vi "FaulhaberV3Communication.vi"(6 "Knoten":u8=1, 7 "Befehl":T1(ring)=enum."SDORead", 8 "error in (no error)":errorcluster, 9 "SendValue":u8[](array[numeric]) format="%02x", 10 "SendObject":u32=1614807040 format="%04x", 11 "VISA resource name":refnum<visa-resource-name>="COM10") -> (0 "error out":errorcluster={"status"=FALSE, "code"=1073676293, "source"="VISA Read in FaulhaberCommunication.vi->Faulhaber_Standalone.vi"}, 1 "Return Value":u8[](array[numeric]) format="%02x", 2 "RecieveObject":u32 format="%08x", 3 "VISA resource name out":refnum<visa-resource-name>="COM10")   [LabVIEW 2011]
panel:
  out "raw":cluster{"unsigned byte array":u8[]}[](array[cluster]) {"unsigned byte array" format="%02x"}
  out "ResponseNo":i32
  out "raw Response":u8[](array[numeric]) format="%02x"
  out "to send unsigned byte array":u8[](array[numeric])=[71, 65, 67, 13] format="%02x"
  out "Bytes send":u32=4
  # "2025 new binary interface"
  # "read with type none"
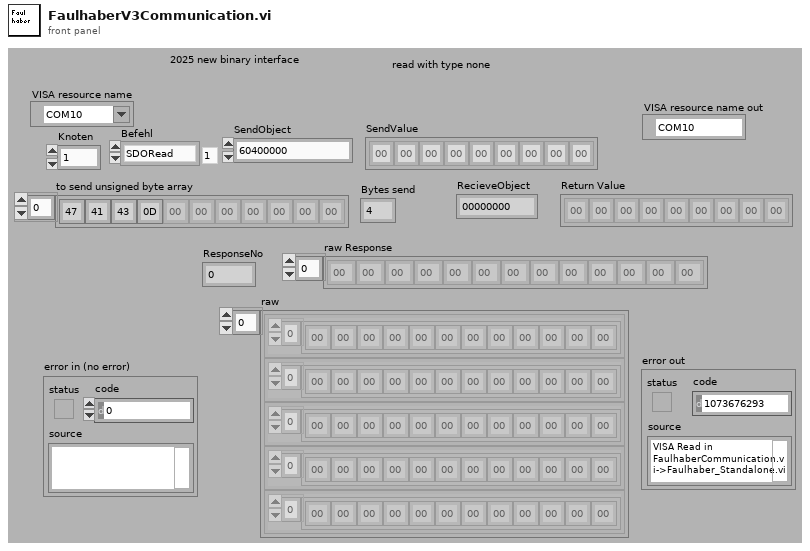
[diagram p1: front panel]
types:
  T1 = enum8{"Bootup", "SDORead", "SDOWrite", "SDOErrror", "Controlword", "Statusword", "TraceLog", "Emcy", "SDOBlockReadInit", "SDOBlockReadUpload", "SDOBlockReadEnd", "SDOBlockWriteInit", "SDOBlockWriteDownload", "SDOBlockWriteEnd"}
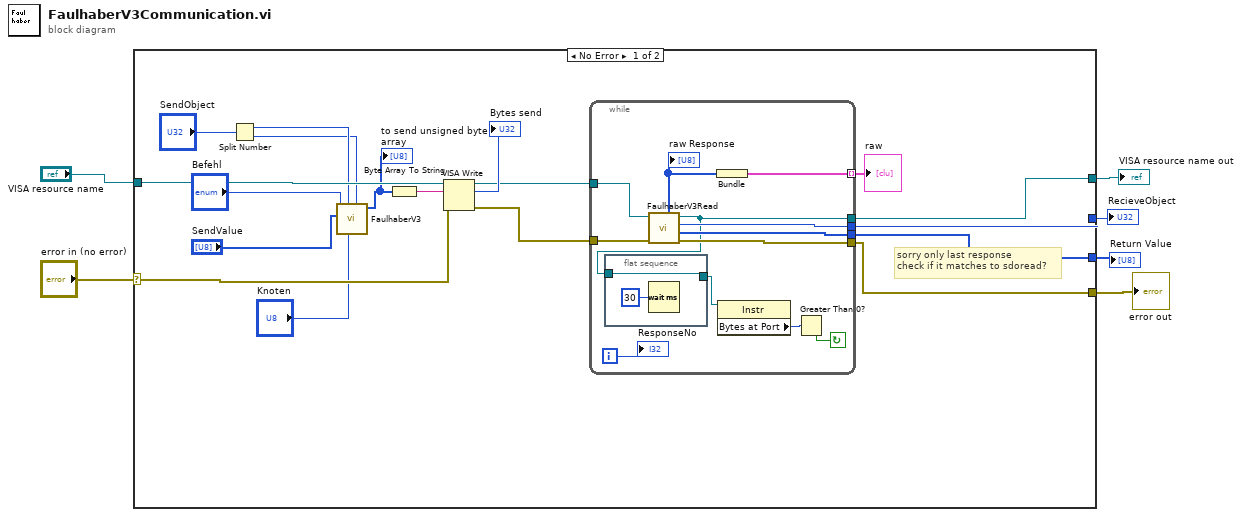
[diagram p0: block diagram]
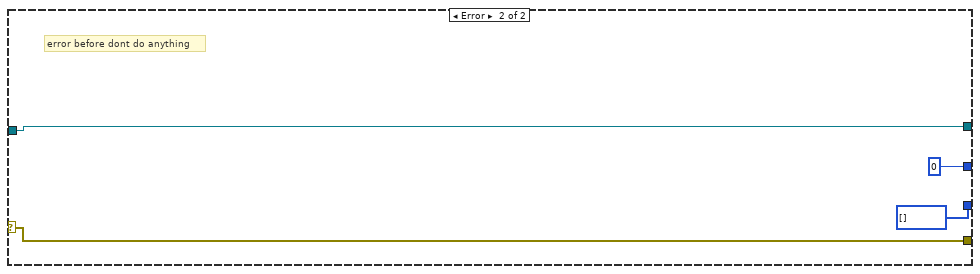
[diagram p2: hidden frame]
diagram:
  n1 = case shown="No Error" "error in (no error)" {
    selector: "error in (no error)" -> [w22 w41]
    tunnel: "VISA resource name" -> [w24 w42]
    tunnel: [w13 w42] -> w5
    tunnel: [w8 w41] -> w4
    tunnel: [w14 u8[] [] ("Value")] -> w1
    tunnel: [w15 u32 0 ("Object")] -> w2
    frame No Error {
      # "sorry only last response\ncheck if it matches to sdoread?"
      n2 = Split Number(x="SendObject") -> (hi(x)=w12:u16, lo(x)=w11:u16)
      n3 = call "FaulhaberV3.vi"("Sub"=w11, "Knoten"="Knoten", "Index"=w12, "SendValue"="SendValue", "Befehl"="Befehl") -> ("Send"=w17:u8[])  [unwired: 6 in]
      "to send unsigned byte array" <- w17
      n4 = Byte Array To String(unsigned byte array=w17) -> (string=w20:string)
      n5 = VISA Write(VISA resource name=w24, write buffer=w20, error in (no error)=w22) -> (VISA resource name out=w16:refnum<visa-resource-name>, return count=→"Bytes send":u32, error out=w9:errorcluster)
      n6 = while {
        tunnel: w16 -> [w36]
        tunnel: [w31] -> w15
        tunnel: [w32] -> w14
        tunnel: [w35] -> w8
        tunnel: [w28] -> w13
        tunnel: w9 -> [w29]
        tunnel: [w25] -> w7 mode=indexing
        i -> [w30]
        stop <- w34 continue-if-true
        n7 = flat-sequence {
          tunnel: w28 -> [w37]
          tunnel: [w37] -> w27
          frame #0 {
            n8 = Wait (ms)(milliseconds to wait=u32 30) -> ()  [unwired: 1 out]
          }
        }
        n9 = call "FaulhaberV3Read.vi"("error in (no error)"=w29, "VISA Refnum in"=w36) -> ("error out"=w35:errorcluster, "Value"=w32:u8[], "Object"=w31:u32, "VISA Refnum out"=w28:refnum<visa-resource-name>, "unsigned byte array"=w26:u8[])  [unwired: 5 in]
        "raw Response" <- w26
        n10 = Bundle("unsigned byte array"=w26) -> (w25:cluster{"unsigned byte array":u8[]})  [unwired: 1 in]
        n11 = property class="Instr"(reference=w27) -> ("Bytes at Port"=w33:u32)  [unwired: 1 in, 2 out]
        n12 = Greater Than 0?(x=w33) -> (x > 0?=w34:bool)
        "ResponseNo" <- w30
      }
      "raw" <- w7
    }
    frame Error {
      # "error before dont do anything"
    }
  }
  "VISA resource name out" <- w5
  "error out" <- w4
  "Return Value" <- w1
  "RecieveObject" <- w2
